vi "MotorControlMina4 with Joystick control.vi"() -> ()   [LabVIEW 2014]
uses:
  <vilib>/Utility/inputDevices.llb/joystickAcquire.vi
  <vilib>/Utility/inputDevices.llb/closeJoystick.vi
  <vilib>/DAQmx/create/channels.llb/DAQmx Create Channel (DO-Digital Output).vi
  <vilib>/DAQmx/write.llb/DAQmx Write (Digital Bool 1Line 1Point).vi
panel:
  in  "Offset (V)":dbl=5.0
  out "Oscillate Mirror? 2":bool
  out "Mirror Voltage":dbl
  in  "Oscillate Mirror?":bool
  in  "Period (s)":i32=1
  in  "Amplitude (V)":dbl=4.0
  in  "Stop":bool
  out "InstrumentMode":T1(ring)=enum."Shutdown"
  in  "XMotorRef":refnum<k7>(container)
  in  "YMotorRef":refnum<k7>(container)
  in  "ZMotorRef":refnum<k7>(container)
  out "JoystOffset":T2={"XOffset"=-99999, "YOffset"=-99999, "ZOffset"=-99999}
  out "RelJoyPos":T3
  in  "InterfaceSelector":T4(tab)
  in  "GoToTopDisp":bool
  in  "GoToBottDisp":bool
  in  "GoToExpLoc":bool
  in  "SaveTopDisp":bool
  in  "SaveBottDisp":bool
  in  "SaveExpLoc":bool
  out "Top Dispenser":T5={"X Pos (mm)"=0.5532008, "Y Pos (mm)"=0.030929338, "Z Pos (mm)"=0.77973413} {"Y Pos (mm)" format="%.3f"; "Z Pos (mm)" format="%.3f"; "X Pos (mm)" format="%.3f"}
  out "Bottom Dispenser":T5={"X Pos (mm)"=0.600309, "Y Pos (mm)"=-1.1540928, "Z Pos (mm)"=0.7938141} {"Y Pos (mm)" format="%.3f"; "Z Pos (mm)" format="%.3f"; "X Pos (mm)" format="%.3f"}
  out "Experiment Region":T5={"X Pos (mm)"=1.4278219, "Y Pos (mm)"=-0.74810517, "Z Pos (mm)"=0.7938141} {"Y Pos (mm)" format="%.3f"; "Z Pos (mm)" format="%.3f"; "X Pos (mm)" format="%.3f"}
  in  "PreviewPanel":T6(tab)
  in  "Z Motor Settings":T7={"Joyst Min Signal"=10.0, "Joyst Max Signal"=30000.0, "Vmax (mm/s)"=0.005, "Acc (mm/s/s)"=0.2, "+ JoystDirection"=2, "- JoystDirection"=1} {"Acc (mm/s/s)" format="%#.3f"; "Vmax (mm/s)" format="%#.3f"}
  in  "Y Motor Settings":T7={"Joyst Min Signal"=10.0, "Joyst Max Signal"=20000.0, "Vmax (mm/s)"=0.03, "Acc (mm/s/s)"=0.5, "+ JoystDirection"=1, "- JoystDirection"=2} {"Acc (mm/s/s)" format="%#.3f"; "Vmax (mm/s)" format="%#.3f"}
  in  "X Motor Settings":T7={"Joyst Min Signal"=10.0, "Joyst Max Signal"=20000.0, "Vmax (mm/s)"=0.03, "Acc (mm/s/s)"=0.5, "+ JoystDirection"=2, "- JoystDirection"=1} {"Acc (mm/s/s)" format="%#.3f"; "Vmax (mm/s)" format="%#.3f"}
  in  "Motor Cruise Param":T8={"X Acc (mm/s^2)"=0.3, "X Vmax (mm/s)"=0.3, "Y Acc (mm/s^2)"=0.3, "Y Vmax (mm/s)"=0.3, "Z Acc (mm/s^2)"=0.1, "Z Vmax (mm/s)"=0.1}
  in  "Motor Limits":T9={"XMin"=-0.8, "XMax"=3.0, "YMin"=-2.0, "YMax"=2.0, "ZMin"=0.0, "ZMax"=2.0}
  in  "Steerable Mirror Calibration":T10={"Hor. Scaling (nm/V)"=760.0, "Vert. Scaling (nm/V)"=760.0, "Hor. Mirr. Offset (V)"=0.0, "Vert. Mirr. Offset (V)"=0.0}
  in  "Steerable \nTrap\n(F12)":bool
  in  "Fixed\nTrap\n(F11)":bool
  in  "Align Traps Vertically":bool
  in  "MaxHorizontalTrapSeparation":bool
  out "X Motor State":T11={"Direction"=0, "Vel (mm/s)"=0.0, "IsActive?"=FALSE, "Pos (mm)"=-0.2957381} {"Pos (mm)" format="%#.3f"; "Vel (mm/s)" format="%#.4f"}
  out "Y Motor State":T11={"Direction"=0, "Vel (mm/s)"=0.0, "IsActive?"=FALSE, "Pos (mm)"=0.016441232} {"Pos (mm)" format="%#.3f"; "Vel (mm/s)" format="%#.4f"}
  out "Z Motor State":T11={"Direction"=0, "Vel (mm/s)"=0.0, "IsActive?"=FALSE, "Pos (mm)"=-0.26253498} {"Pos (mm)" format="%#.3f"; "Vel (mm/s)" format="%#.4f"}
  out "Move Z":bool
  out "Move XY":bool
  in  "MotorLoopDelay":u32=100
  in  "StopPassiveMode":bool caption="stop"
  in  "PMVertSlider(V)":dbl(slide)=0.005145263671875 scale=0.0..10.0 scale format="%#_3f"
  in  "PMHorizSlider(V)":dbl(slide)=0.0045623779296875 scale=2.0..10.0
  out "IsPassiveModeActive?":bool caption="stop"
  out "Force TrapA":cluster{"x":dbl[], "y":dbl[]}[](graph)
  out "Noise-Ext":cluster{"x":dbl[], "y":dbl[]}[](graph)
  out "Force TrapB":cluster{"x":dbl[], "y":dbl[]}[](graph)
  out "IsOffsetModeActive?":bool caption="stop"
  in  "StopOffset":bool caption="stop"
  out "IsForceExtActive?":bool=TRUE
  in  "StopForceExtension":bool caption="stop"
  # "ClpXP Optical Tweezers"
  # "Chamber Locations"
  # "Need a Button Here that would read the \nNormalized Offset and save it"
  # "Off"
  # "On"
  # "Off"
  # "On"
  # "Thorlabs Motor Status"
  # "Passive Mode"
  # "when I switch tabs from the passive mode to basic mode, the recording doesn't stop"
  # "The sliders don't do anything in passive mode, fix it"
  # "Whenever I click on Ackquire Offset, it goes back to the basic operation, then I have to ckick again"
  # "Trap Motion Control"
  # "Steerable Mirror Info"
  # "Zero-Force Offset Mode"
  # "High Frequency Data Acquisition"
  # "Adjust the length of acquisition time"
  # "Force-Extension Mode"
  # "Y"
  # "+"
  # "X"
  # "-"
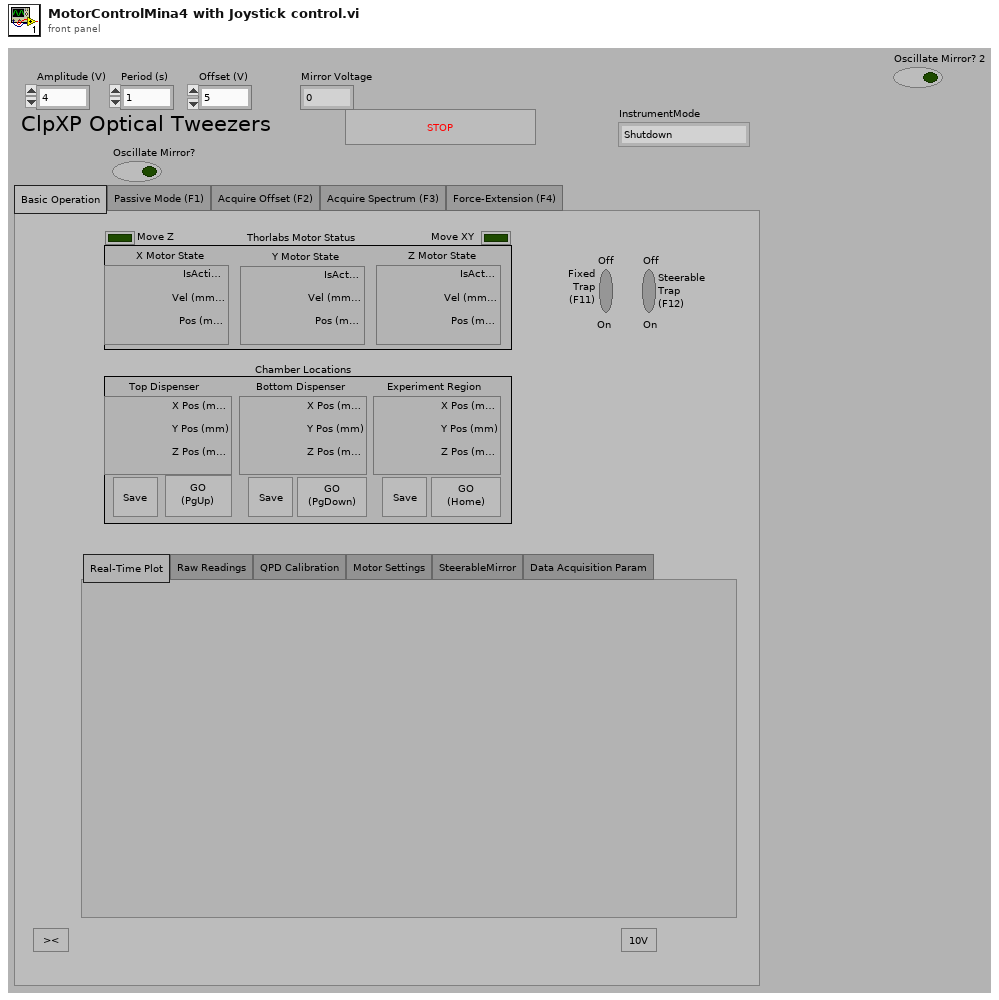
[diagram p1: front panel]
types:
  T1 = enum16{"InitializeJoystick", "InitializeMotors", "BasicMode", "PassiveMode", "AcquireOffsetMode", "AcquireSpectrumMode", "Force-ExtensionMode", "Shutdown"}
  T2 = cluster{"XOffset":i32, "YOffset":i32, "ZOffset":i32}
  T3 = cluster{"XRelPos":i32, "YRelPos":i32, "ZRelPos":i32}
  T4 = enum32{"Basic Operation", "Passive Mode (F1)", "Acquire Offset (F2)", "Acquire Spectrum (F3)", "Force-Extension (F4)"}
  T5 = cluster{"X Pos (mm)":sgl, "Y Pos (mm)":sgl, "Z Pos (mm)":sgl}
  T6 = enum32{"Real-Time Plot", "Raw Readings", "QPD Calibration", "Motor Settings", "SteerableMirror", "Data Acquisition Param"}
  T7 = cluster{"Joyst Min Signal":dbl, "Joyst Max Signal":dbl, "Vmax (mm/s)":sgl, "Acc (mm/s/s)":sgl, "+ JoystDirection":i32, "- JoystDirection":i32}
  T8 = cluster{"X Acc (mm/s^2)":sgl, "X Vmax (mm/s)":sgl, "Y Acc (mm/s^2)":sgl, "Y Vmax (mm/s)":sgl, "Z Acc (mm/s^2)":sgl, "Z Vmax (mm/s)":sgl}
  T9 = cluster{"XMin":sgl, "XMax":sgl, "YMin":sgl, "YMax":sgl, "ZMin":sgl, "ZMax":sgl}
  T10 = cluster{"Hor. Scaling (nm/V)":dbl, "Vert. Scaling (nm/V)":dbl, "Hor. Mirr. Offset (V)":dbl, "Vert. Mirr. Offset (V)":dbl}
  T11 = cluster{"Direction":i32, "Vel (mm/s)":sgl, "IsActive?":bool, "Pos (mm)":sgl}
  T12 = cluster{"XMotorRef":refnum<k7>, "YMotorRef":refnum<k7>, "ZMotorRef":refnum<k7>}
  T13 = cluster{"Motor Reference":refnum<k7>, "Motor Reference":refnum<k7>, "Motor Reference":refnum<k7>}
  T14 = cluster{"X axis":i32, "Y axis":i32, "Z axis":i32, "X axis rotation":i32, "Y axis rotation":i32, "Z axis rotation":i32, "U axis":i32, "V axis":i32}
  T15 = cluster{"button 1":bool, "button 2":bool, "button 3":bool, "button 4":bool, "button 5":bool, "button 6":bool, "button 7":bool, "button 8":bool, "button 9":bool, "button 10":bool, "button 11":bool, "button 12":bool, "button 13":bool, "button 14":bool, "button 15":bool, "button 16":bool, "button 17":bool, "button 18":bool, "button 19":bool, "button 20":bool, "button 21":bool, "button 22":bool, "button 23":bool, "button 24":bool, "button 25":bool, "button 26":bool, "button 27":bool, "button 28":bool, "button 29":bool, "button 30":bool, "button 31":bool, "button 32":bool}
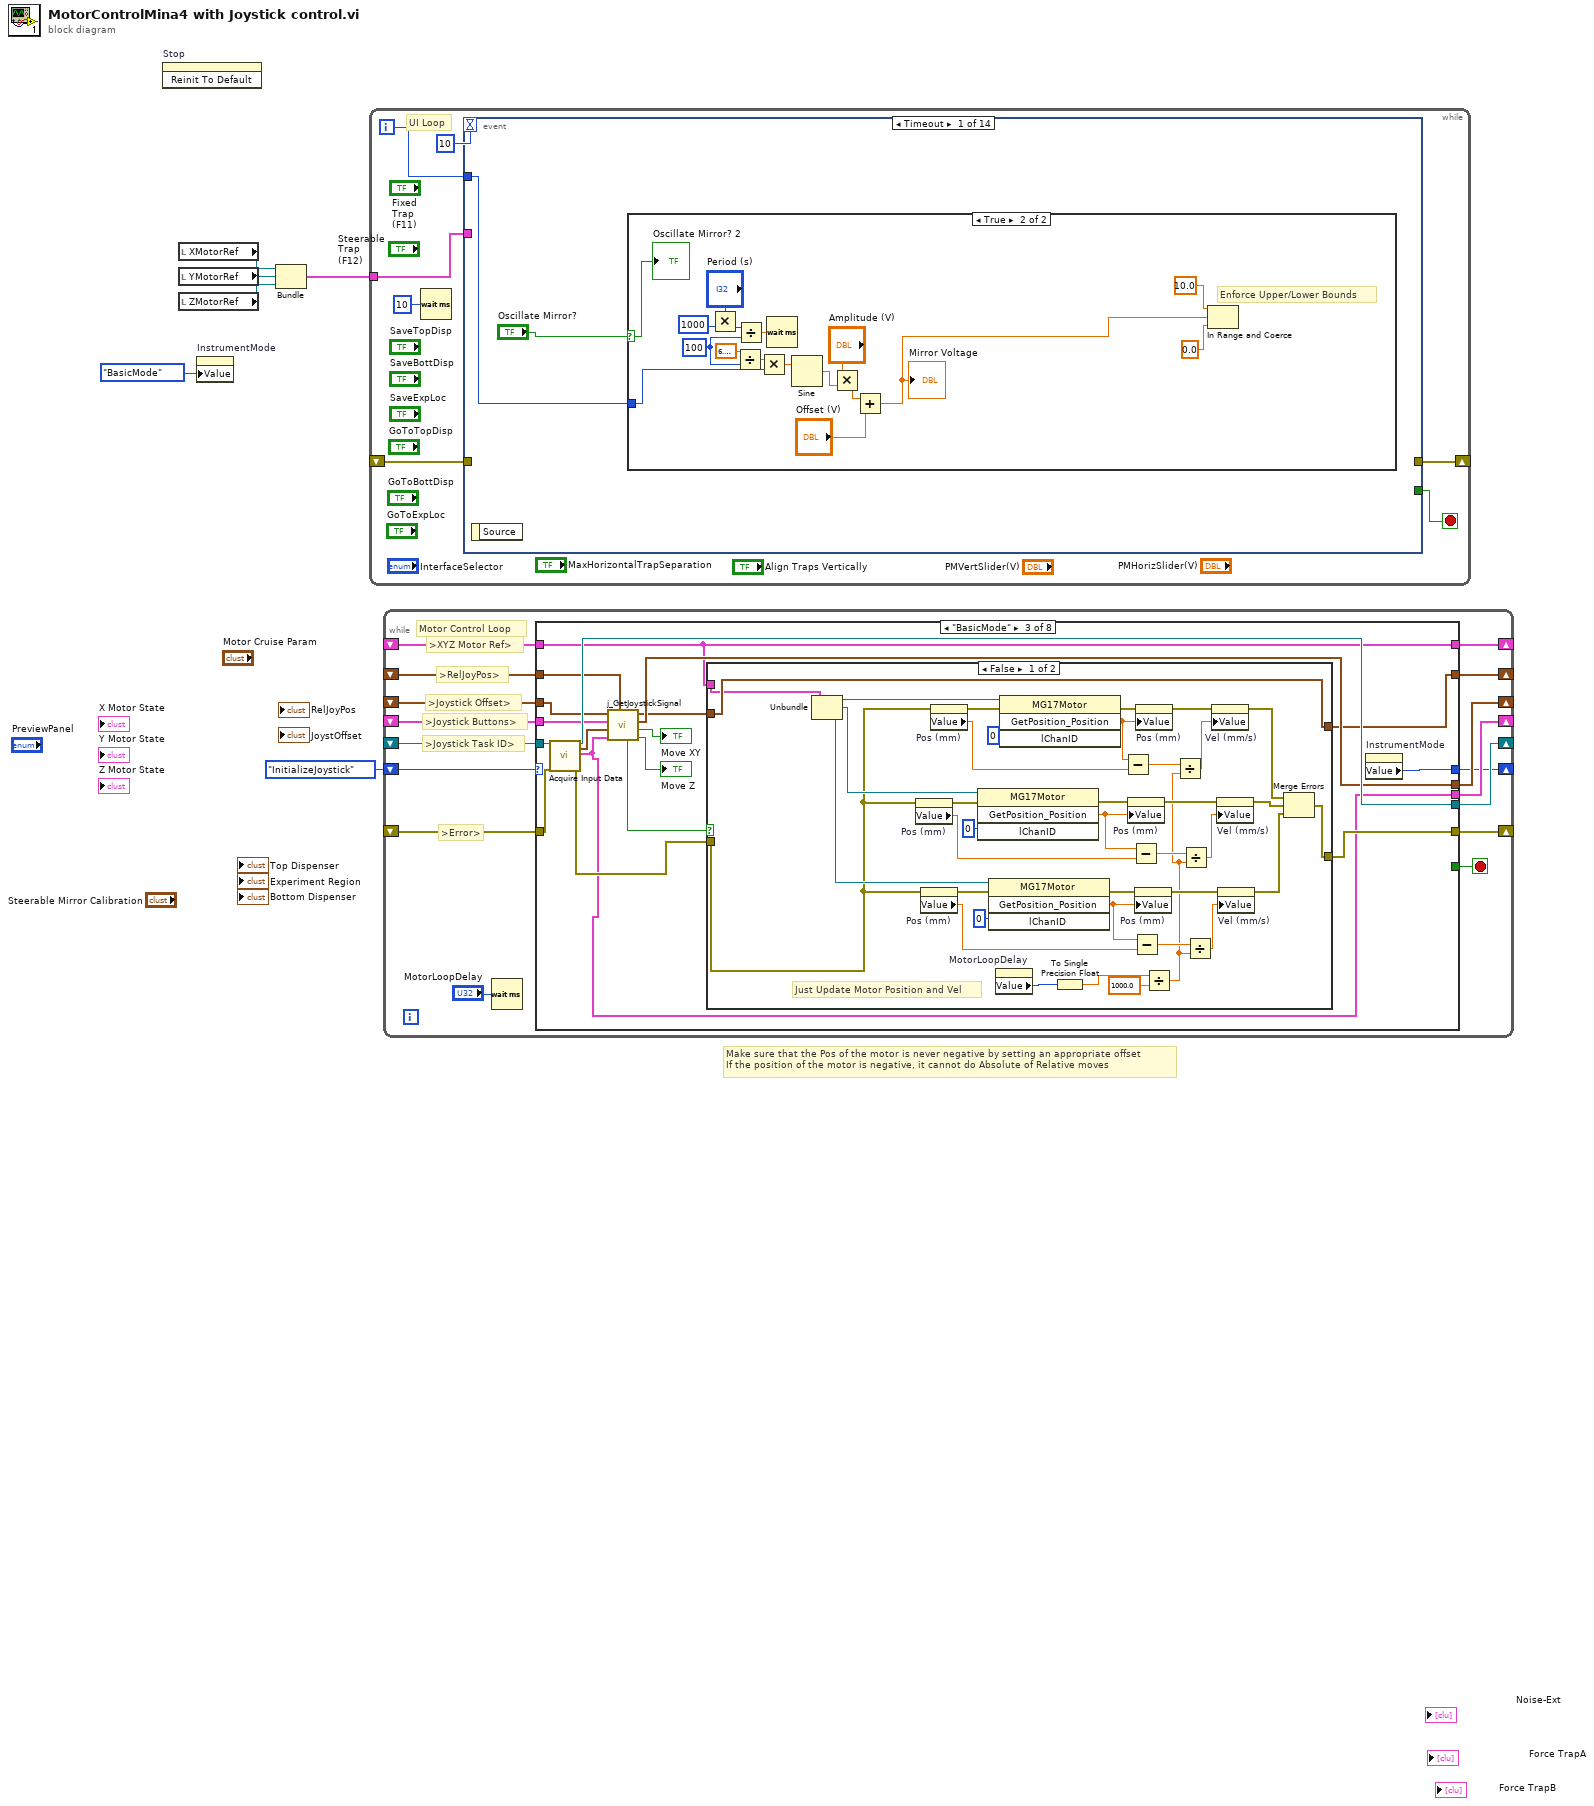
[diagram p0: block diagram]
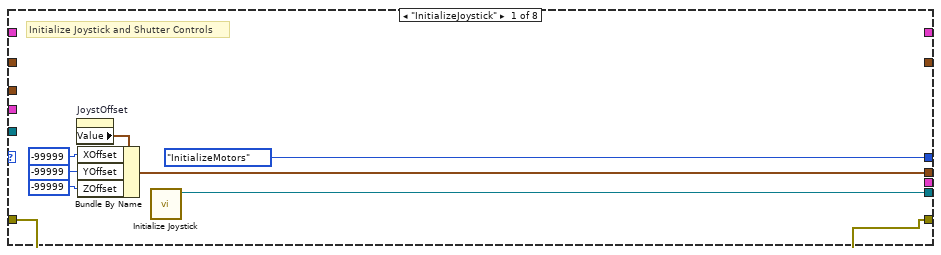
[diagram p2: hidden frame]
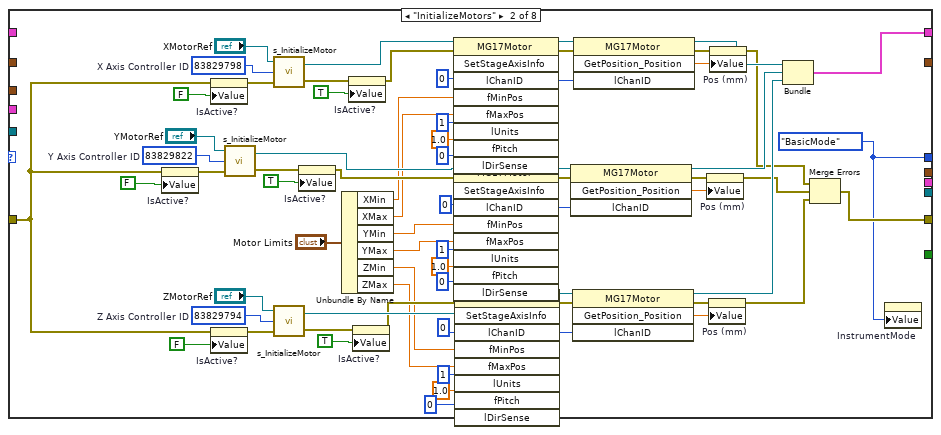
[diagram p3: hidden frame]
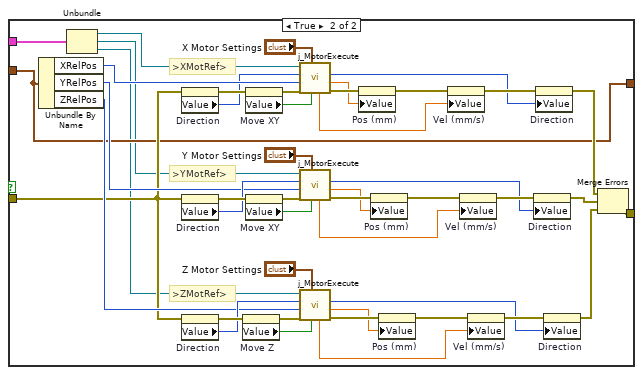
[diagram p4: hidden frame]
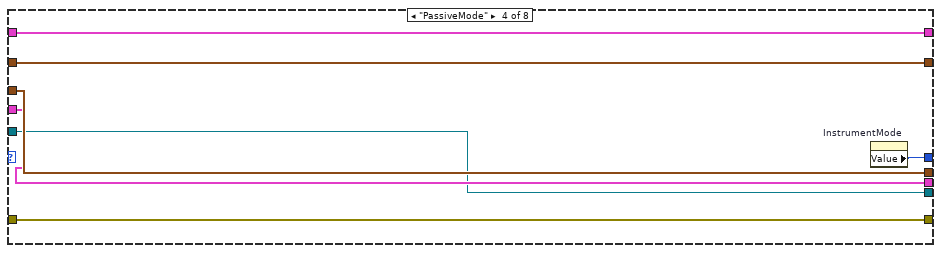
[diagram p5: hidden frame]
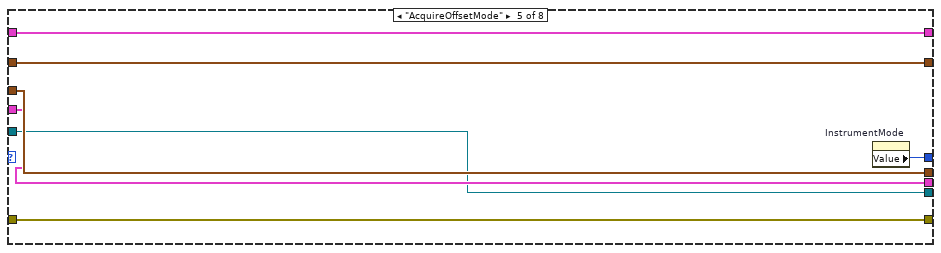
[diagram p6: hidden frame]
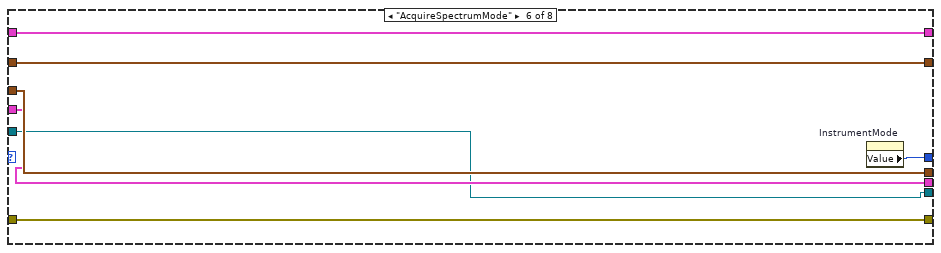
[diagram p7: hidden frame]
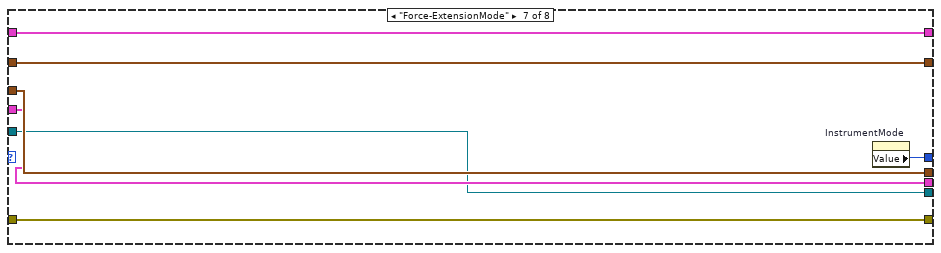
[diagram p8: hidden frame]
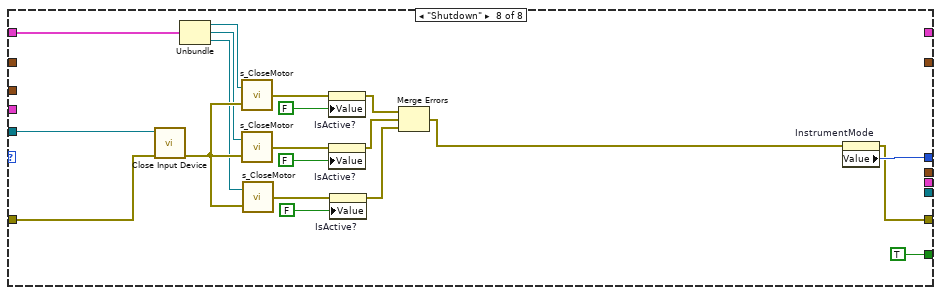
[diagram p9: hidden frame]
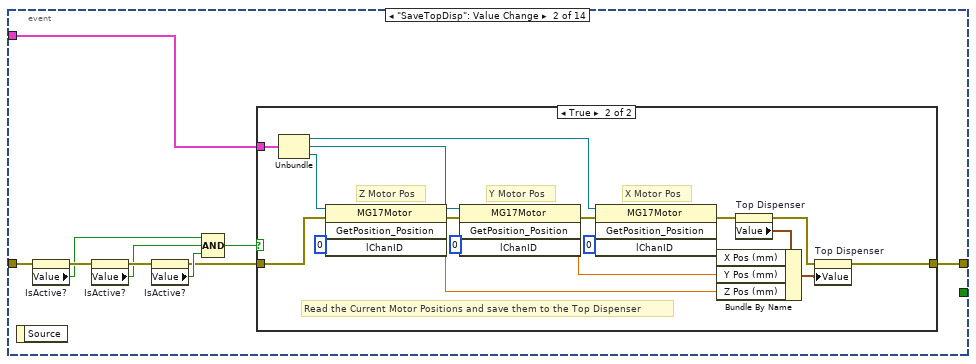
[diagram p11: hidden frame]
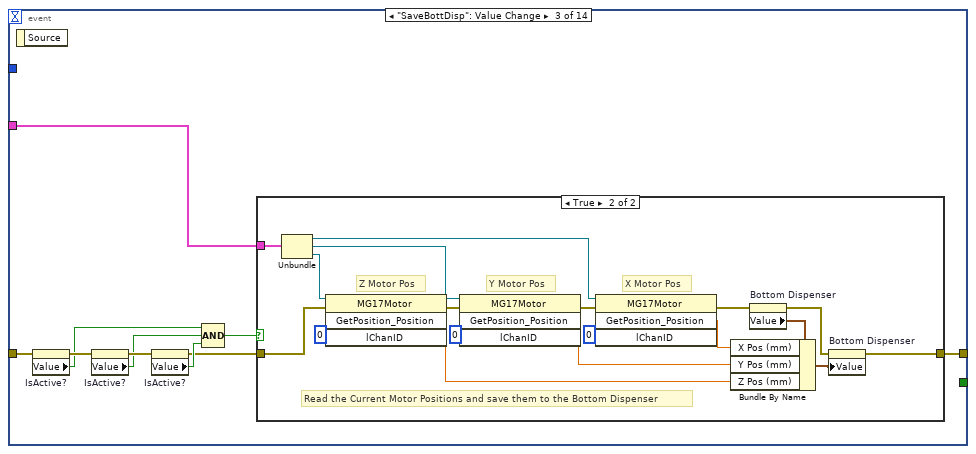
[diagram p13: hidden frame]
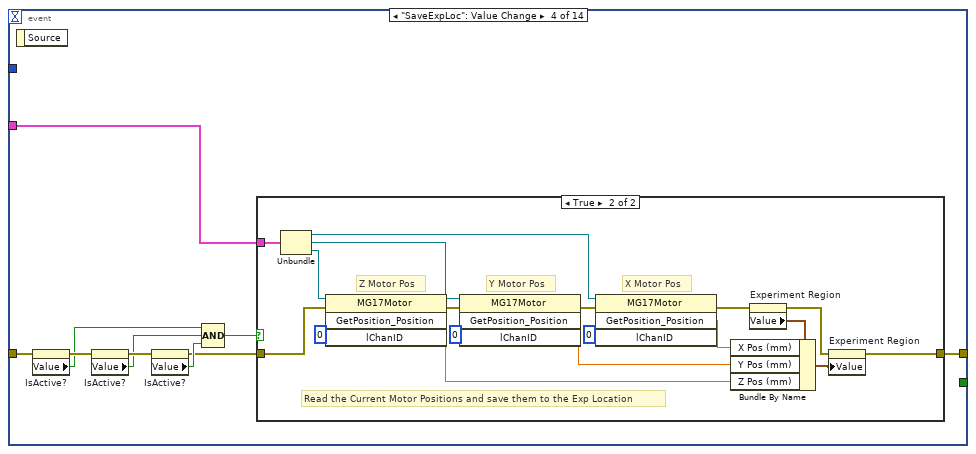
[diagram p15: hidden frame]
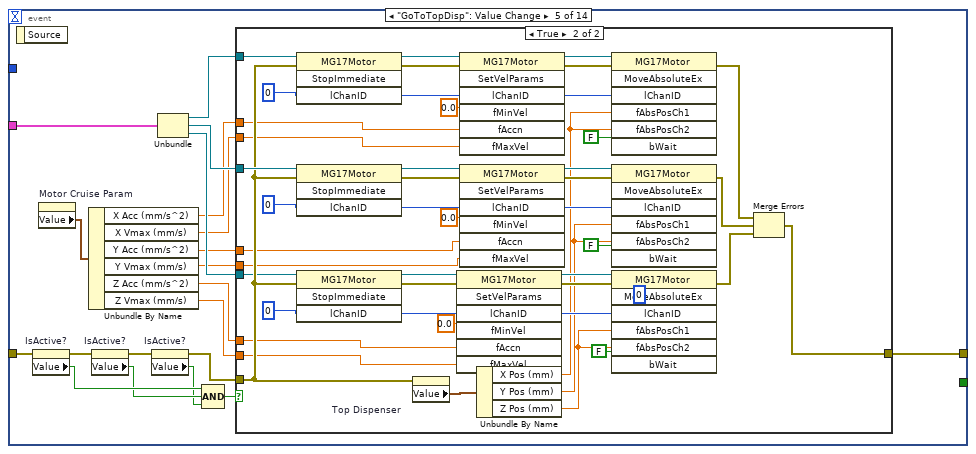
[diagram p17: hidden frame]
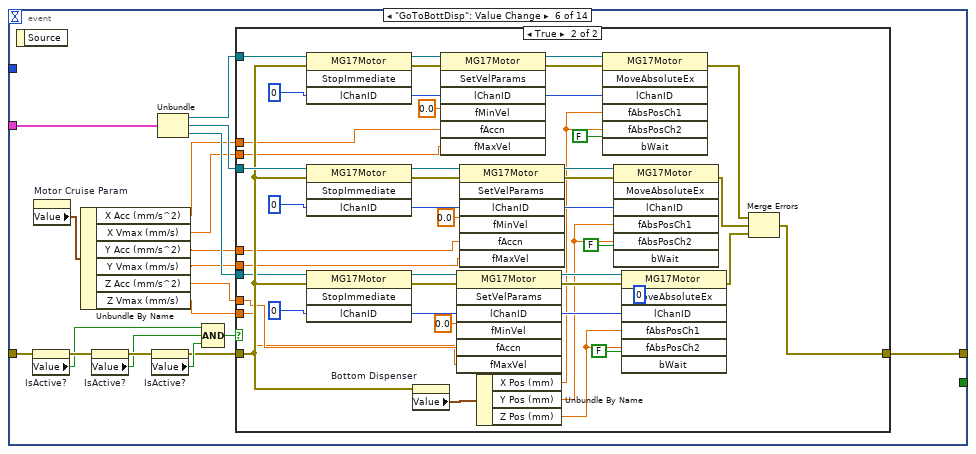
[diagram p19: hidden frame]
diagram:
  # "Make sure that the Pos of the motor is never negative by setting an appropriate offset\nIf the position of the motor is negative, it cannot do Absolute of Relative moves"
  n1 = invoke on="Stop" class="Bool" method="Reinit To Default"() -> ()  [unwired: 3 in, 3 out]
  n2 = local read "XMotorRef"() -> (w6:refnum<k7>)
  n3 = local read "YMotorRef"() -> (w5:refnum<k7>)
  n4 = local read "ZMotorRef"() -> (w4:refnum<k7>)
  n5 = property on="InstrumentMode" class="Enum (strict)"("Value"=T1."BasicMode") -> ()  [unwired: 2 in, 2 out]
  n6 = Bundle("XMotorRef"=w6, "YMotorRef"=w5, "ZMotorRef"=w4) -> (w3:T12)  [unwired: 1 in]
  n7 = while {
    shift-right: [w12] -> _
    shift-left: _ -> [w11]
    tunnel: w3 -> [w10]
    i -> [w8]
    stop <- w9 stop-if-true
    # "UI Loop"
    n8 = Wait (ms)(milliseconds to wait=u32 10) -> ()  [unwired: 1 out]
    n9 = event shown="[0] Timeout" {
      selector: _ -> [_ _ _ _ _ _ _ _ _ _ _ _ _ _]
      dyn-events: _ -> [_ _ _ _ _ _ _ _ _ _ _ _ _ _]
      timeout: 10 -> [_ _ _ _ _ _ _ _ _ _ _ _ _ _]
      tunnel: [_ w35 w64 w93 w132 w198 w264 w318 _ w329 _ _ _ w357] -> w12
      tunnel: w11 -> [_ w34 w63 w92 w131 w197 w263 w321 w328 w329 _ _ _ w357]
      tunnel: [_ _ _ _ _ _ _ _ _ _ _ _ _ "Stop"] -> w9
      tunnel: w10 -> [_ w33 w62 w91 w130 w196 w262 _ _ _ _ _ _ _]
      tunnel: w8 -> [w15 _ _ _ _ _ _ _ _ _ _ _ _ _]
      tunnel: [_ _ _ _ _ _ _ _ w328 _ _ _ _ _] -> _
      event Timeout {
        n10 = event-data() -> ()  [unwired: 1 in, 1 out]
        n11 = case shown="True" "Oscillate Mirror?" {
          selector: "Oscillate Mirror?" -> [_ w21]
          tunnel: w15 -> [_ w22]
          frame False {
          }
          frame True {
            w31 = 100
            # "Enforce Upper/Lower Bounds"
            n12 = Multiply(x="Period (s)", y=1000) -> (x*y=w29:i32)
            n13 = Divide(x=6.283185307179586, y=w31) -> (x/y=w25:dbl)
            n14 = Divide(x=w29, y=w31) -> (x/y=w30:dbl)
            n15 = Multiply(x=w25, y=w22) -> (x*y=w26:dbl)
            n16 = Wait (ms)(milliseconds to wait=w30) -> ()  [unwired: 1 out]
            n17 = Sine(x=w26) -> (sin(x)=w27:dbl)
            n18 = Multiply(x="Amplitude (V)", y=w27) -> (x*y=w19:dbl)
            n19 = Add(x=w19, y="Offset (V)") -> (x+y=w16:dbl)
            "Mirror Voltage" <- w16
            n20 = In Range and Coerce(upper limit=10.0, x=w16, lower limit=0.0 ("upper limit")) -> ()  [unwired: 2 out]
            "Oscillate Mirror? 2" <- w21
          }
        }
      }
      event "SaveTopDisp": Value Change {
        n21 = event-data() -> ()  [unwired: 1 in, 1 out]
        n22 = property on="IsActive?" class="Bool (strict)"(error in=w34) -> (error out=w42:errorcluster, "Value"=w40:bool)  [unwired: 1 in, 1 out]
        n23 = property on="IsActive?" class="Bool (strict)"(error in=w42) -> (error out=w41:errorcluster, "Value"=w39:bool)  [unwired: 1 in, 1 out]
        n24 = property on="IsActive?" class="Bool (strict)"(error in=w41) -> (error out=w36:errorcluster, "Value"=w38:bool)  [unwired: 1 in, 1 out]
        n25 = Compound Arithmetic op=AND(w40, w39, w38) -> (w37:bool)
        n26 = case shown="True" w37 {
          tunnel: w36 -> [w43 w61]
          tunnel: [w43 w48] -> w35
          tunnel: w33 -> [_ w47]
          frame False {
          }
          frame True {
            # "Read the Current Motor Positions and save them to the Top Dispenser"
            # "X Motor Pos"
            # "Y Motor Pos"
            # "Z Motor Pos"
            n27 = Unbundle(w47) -> ("XMotorRef"=w44:refnum<k7>, "YMotorRef"=w45:refnum<k7>, "ZMotorRef"=w46:refnum<k7>)
            n28 = invoke class="MG17Motor" method="GetPosition_Position"(reference=w46, error in=w61, "lChanID"=0) -> (error out=w58:errorcluster, "GetPosition_Position"=w51:sgl)  [unwired: 1 in, 2 out]
            n29 = invoke class="MG17Motor" method="GetPosition_Position"(reference=w45, error in=w58, "lChanID"=0) -> (error out=w56:errorcluster, "GetPosition_Position"=w50:sgl)  [unwired: 1 in, 2 out]
            n30 = invoke class="MG17Motor" method="GetPosition_Position"(reference=w44, error in=w56, "lChanID"=0) -> (error out=w55:errorcluster, "GetPosition_Position"=w49:sgl)  [unwired: 1 in, 2 out]
            n31 = property on="Top Dispenser" class="Clust (strict)"(error in=w55) -> (error out=w54:errorcluster, "Value"=w53:T5)  [unwired: 1 in, 1 out]
            n32 = Bundle By Name(cluster=w53, "X Pos (mm)"=w49, "Y Pos (mm)"=w50, "Z Pos (mm)"=w51) -> (w52:T5)
            n33 = property on="Top Dispenser" class="Clust (strict)"(error in=w54, "Value"=w52) -> (error out=w48:errorcluster)  [unwired: 1 in, 1 out]
          }
        }
      }
      event "SaveBottDisp": Value Change {
        n34 = event-data() -> ()  [unwired: 1 in, 1 out]
        n35 = property on="IsActive?" class="Bool (strict)"(error in=w63) -> (error out=w71:errorcluster, "Value"=w69:bool)  [unwired: 1 in, 1 out]
        n36 = property on="IsActive?" class="Bool (strict)"(error in=w71) -> (error out=w70:errorcluster, "Value"=w68:bool)  [unwired: 1 in, 1 out]
        n37 = property on="IsActive?" class="Bool (strict)"(error in=w70) -> (error out=w65:errorcluster, "Value"=w67:bool)  [unwired: 1 in, 1 out]
        n38 = Compound Arithmetic op=AND(w69, w68, w67) -> (w66:bool)
        n39 = case shown="True" w66 {
          tunnel: w65 -> [w72 w90]
          tunnel: [w72 w77] -> w64
          tunnel: w62 -> [_ w76]
          frame False {
          }
          frame True {
            # "Read the Current Motor Positions and save them to the Bottom Dispenser"
            # "X Motor Pos"
            # "Y Motor Pos"
            # "Z Motor Pos"
            n40 = Unbundle(w76) -> ("XMotorRef"=w73:refnum<k7>, "YMotorRef"=w74:refnum<k7>, "ZMotorRef"=w75:refnum<k7>)
            n41 = invoke class="MG17Motor" method="GetPosition_Position"(reference=w75, error in=w90, "lChanID"=0) -> (error out=w87:errorcluster, "GetPosition_Position"=w80:sgl)  [unwired: 1 in, 2 out]
            n42 = invoke class="MG17Motor" method="GetPosition_Position"(reference=w74, error in=w87, "lChanID"=0) -> (error out=w85:errorcluster, "GetPosition_Position"=w79:sgl)  [unwired: 1 in, 2 out]
            n43 = invoke class="MG17Motor" method="GetPosition_Position"(reference=w73, error in=w85, "lChanID"=0) -> (error out=w84:errorcluster, "GetPosition_Position"=w78:sgl)  [unwired: 1 in, 2 out]
            n44 = property on="Bottom Dispenser" class="Clust (strict)"(error in=w84) -> (error out=w83:errorcluster, "Value"=w82:T5)  [unwired: 1 in, 1 out]
            n45 = Bundle By Name(cluster=w82, "X Pos (mm)"=w78, "Y Pos (mm)"=w79, "Z Pos (mm)"=w80) -> (w81:T5)
            n46 = property on="Bottom Dispenser" class="Clust (strict)"(error in=w83, "Value"=w81) -> (error out=w77:errorcluster)  [unwired: 1 in, 1 out]
          }
        }
      }
      event "SaveExpLoc": Value Change {
        n47 = event-data() -> ()  [unwired: 1 in, 1 out]
        n48 = property on="IsActive?" class="Bool (strict)"(error in=w92) -> (error out=w100:errorcluster, "Value"=w98:bool)  [unwired: 1 in, 1 out]
        n49 = property on="IsActive?" class="Bool (strict)"(error in=w100) -> (error out=w99:errorcluster, "Value"=w97:bool)  [unwired: 1 in, 1 out]
        n50 = property on="IsActive?" class="Bool (strict)"(error in=w99) -> (error out=w94:errorcluster, "Value"=w96:bool)  [unwired: 1 in, 1 out]
        n51 = Compound Arithmetic op=AND(w98, w97, w96) -> (w95:bool)
        n52 = case shown="True" w95 {
          tunnel: w94 -> [w101 w119]
          tunnel: [w101 w106] -> w93
          tunnel: w91 -> [_ w105]
          frame False {
          }
          frame True {
            # "Read the Current Motor Positions and save them to the Exp Location"
            # "X Motor Pos"
            # "Y Motor Pos"
            # "Z Motor Pos"
            n53 = Unbundle(w105) -> ("XMotorRef"=w102:refnum<k7>, "YMotorRef"=w103:refnum<k7>, "ZMotorRef"=w104:refnum<k7>)
            n54 = invoke class="MG17Motor" method="GetPosition_Position"(reference=w104, error in=w119, "lChanID"=0) -> (error out=w116:errorcluster, "GetPosition_Position"=w109:sgl)  [unwired: 1 in, 2 out]
            n55 = invoke class="MG17Motor" method="GetPosition_Position"(reference=w103, error in=w116, "lChanID"=0) -> (error out=w114:errorcluster, "GetPosition_Position"=w108:sgl)  [unwired: 1 in, 2 out]
            n56 = invoke class="MG17Motor" method="GetPosition_Position"(reference=w102, error in=w114, "lChanID"=0) -> (error out=w113:errorcluster, "GetPosition_Position"=w107:sgl)  [unwired: 1 in, 2 out]
            n57 = property on="Experiment Region" class="Clust (strict)"(error in=w113) -> (error out=w112:errorcluster, "Value"=w111:T5)  [unwired: 1 in, 1 out]
            n58 = Bundle By Name(cluster=w111, "X Pos (mm)"=w107, "Y Pos (mm)"=w108, "Z Pos (mm)"=w109) -> (w110:T5)
            n59 = property on="Experiment Region" class="Clust (strict)"(error in=w112, "Value"=w110) -> (error out=w106:errorcluster)  [unwired: 1 in, 1 out]
          }
        }
      }
      event "GoToTopDisp": Value Change {
        n60 = event-data() -> ()  [unwired: 1 in, 1 out]
        n61 = property on="IsActive?" class="Bool (strict)"(error in=w131) -> (error out=w139:errorcluster, "Value"=w137:bool)  [unwired: 1 in, 1 out]
        n62 = property on="Motor Cruise Param" class="Clust (strict)"() -> ("Value"=w120:T8)  [unwired: 2 in, 2 out]
        n63 = Unbundle By Name(w120) -> ("X Acc (mm/s^2)"=w124:sgl, "X Vmax (mm/s)"=w123:sgl, "Y Acc (mm/s^2)"=w122:sgl, "Y Vmax (mm/s)"=w121:sgl, "Z Acc (mm/s^2)"=w126:sgl, "Z Vmax (mm/s)"=w125:sgl)
        n64 = property on="IsActive?" class="Bool (strict)"(error in=w139) -> (error out=w138:errorcluster, "Value"=w136:bool)  [unwired: 1 in, 1 out]
        n65 = property on="IsActive?" class="Bool (strict)"(error in=w138) -> (error out=w133:errorcluster, "Value"=w135:bool)  [unwired: 1 in, 1 out]
        n66 = Unbundle(w130) -> ("XMotorRef"=w129:refnum<k7>, "YMotorRef"=w128:refnum<k7>, "ZMotorRef"=w127:refnum<k7>)
        n67 = Compound Arithmetic op=AND(w137, w136, w135) -> (w134:bool)
        n68 = case shown="True" w134 {
          tunnel: w133 -> [w140 w160]
          tunnel: [w140 w156] -> w132
          tunnel: w129 -> [_ w183]
          tunnel: w128 -> [_ w168]
          tunnel: w127 -> [_ w155]
          tunnel: w126 -> [_ w146]
          tunnel: w125 -> [_ w145]
          tunnel: w124 -> [_ w144]
          tunnel: w123 -> [_ w143]
          tunnel: w122 -> [_ w142]
          tunnel: w121 -> [_ w141]
          frame False {
          }
          frame True {
            (unwired) 0 ("lChanID")
            n69 = invoke class="MG17Motor" method="StopImmediate"(reference=w183, error in=w160, "lChanID"=0) -> (reference out=w181:refnum<k7>, error out=w182:errorcluster, "lChanID"=w151:i32)  [unwired: 1 in, 1 out]
            n70 = invoke class="MG17Motor" method="StopImmediate"(reference=w168, error in=w160, "lChanID"=0) -> (reference out=w175:refnum<k7>, error out=w176:errorcluster, "lChanID"=w152:i32)  [unwired: 1 in, 1 out]
            n71 = invoke class="MG17Motor" method="StopImmediate"(reference=w155, error in=w160, "lChanID"=0) -> (reference out=w165:refnum<k7>, error out=w166:errorcluster, "lChanID"=w153:i32)  [unwired: 1 in, 1 out]
            n72 = property on="Top Dispenser" class="Clust (strict)"(error in=w160) -> ("Value"=w185:T5)  [unwired: 1 in, 2 out]
            n73 = invoke class="MG17Motor" method="SetVelParams"(reference=w165, error in=w166, "lChanID"=w153, "fMinVel"=sgl 0.0, "fAccn"=w146, "fMaxVel"=w145) -> (reference out=w164:refnum<k7>, error out=w163:errorcluster, "lChanID"=w162:i32)  [unwired: 1 in, 4 out]
            n74 = invoke class="MG17Motor" method="SetVelParams"(reference=w181, error in=w182, "lChanID"=w151, "fMinVel"=sgl 0.0, "fAccn"=w144, "fMaxVel"=w143) -> (reference out=w180:refnum<k7>, error out=w179:errorcluster, "lChanID"=w178:i32)  [unwired: 1 in, 4 out]
            n75 = invoke class="MG17Motor" method="SetVelParams"(reference=w175, error in=w176, "lChanID"=w152, "fMinVel"=sgl 0.0, "fAccn"=w142, "fMaxVel"=w141) -> (reference out=w173:refnum<k7>, error out=w172:errorcluster, "lChanID"=w171:i32)  [unwired: 1 in, 4 out]
            n76 = Unbundle By Name(w185) -> ("X Pos (mm)"=w149:sgl, "Y Pos (mm)"=w148:sgl, "Z Pos (mm)"=w147:sgl)
            n77 = invoke class="MG17Motor" method="MoveAbsoluteEx"(reference=w180, error in=w179, "lChanID"=w178, "fAbsPosCh1"=w149, "fAbsPosCh2"=w149, "bWait"=FALSE) -> (error out=w159:errorcluster)  [unwired: 1 in, 6 out]
            n78 = invoke class="MG17Motor" method="MoveAbsoluteEx"(reference=w173, error in=w172, "lChanID"=w171, "fAbsPosCh1"=w148, "fAbsPosCh2"=w148, "bWait"=FALSE) -> (error out=w158:errorcluster)  [unwired: 1 in, 6 out]
            n79 = invoke class="MG17Motor" method="MoveAbsoluteEx"(reference=w164, error in=w163, "lChanID"=w162, "fAbsPosCh1"=w147, "fAbsPosCh2"=w147, "bWait"=FALSE) -> (error out=w157:errorcluster)  [unwired: 1 in, 6 out]
            n80 = Merge Errors(w159, w158, w157) -> (w156:errorcluster)
          }
        }
      }
      event "GoToBottDisp": Value Change {
        n81 = event-data() -> ()  [unwired: 1 in, 1 out]
        n82 = property on="IsActive?" class="Bool (strict)"(error in=w197) -> (error out=w205:errorcluster, "Value"=w203:bool)  [unwired: 1 in, 1 out]
        n83 = property on="Motor Cruise Param" class="Clust (strict)"() -> ("Value"=w192:T8)  [unwired: 2 in, 2 out]
        n84 = Unbundle By Name(w192) -> ("X Acc (mm/s^2)"=w191:sgl, "X Vmax (mm/s)"=w190:sgl, "Y Acc (mm/s^2)"=w189:sgl, "Y Vmax (mm/s)"=w188:sgl, "Z Acc (mm/s^2)"=w187:sgl, "Z Vmax (mm/s)"=w186:sgl)
        n85 = property on="IsActive?" class="Bool (strict)"(error in=w205) -> (error out=w204:errorcluster, "Value"=w202:bool)  [unwired: 1 in, 1 out]
        n86 = property on="IsActive?" class="Bool (strict)"(error in=w204) -> (error out=w199:errorcluster, "Value"=w201:bool)  [unwired: 1 in, 1 out]
        n87 = Unbundle(w196) -> ("XMotorRef"=w195:refnum<k7>, "YMotorRef"=w194:refnum<k7>, "ZMotorRef"=w193:refnum<k7>)
        n88 = Compound Arithmetic op=AND(w203, w202, w201) -> (w200:bool)
        n89 = case shown="True" w200 {
          tunnel: w199 -> [w206 w226]
          tunnel: [w206 w222] -> w198
          tunnel: w195 -> [_ w249]
          tunnel: w194 -> [_ w234]
          tunnel: w193 -> [_ w221]
          tunnel: w191 -> [_ w212]
          tunnel: w190 -> [_ w211]
          tunnel: w189 -> [_ w210]
          tunnel: w188 -> [_ w209]
          tunnel: w187 -> [_ w208]
          tunnel: w186 -> [_ w207]
          frame False {
          }
          frame True {
            (unwired) 0 ("lChanID")
            n90 = invoke class="MG17Motor" method="StopImmediate"(reference=w249, error in=w226, "lChanID"=0) -> (reference out=w247:refnum<k7>, error out=w248:errorcluster, "lChanID"=w217:i32)  [unwired: 1 in, 1 out]
            n91 = invoke class="MG17Motor" method="StopImmediate"(reference=w234, error in=w226, "lChanID"=0) -> (reference out=w241:refnum<k7>, error out=w242:errorcluster, "lChanID"=w218:i32)  [unwired: 1 in, 1 out]
            n92 = invoke class="MG17Motor" method="StopImmediate"(reference=w221, error in=w226, "lChanID"=0) -> (reference out=w231:refnum<k7>, error out=w232:errorcluster, "lChanID"=w219:i32)  [unwired: 1 in, 1 out]
            n93 = property on="Bottom Dispenser" class="Clust (strict)"(error in=w226) -> ("Value"=w251:T5)  [unwired: 1 in, 2 out]
            n94 = invoke class="MG17Motor" method="SetVelParams"(reference=w247, error in=w248, "lChanID"=w217, "fMinVel"=sgl 0.0, "fAccn"=w212, "fMaxVel"=w211) -> (reference out=w246:refnum<k7>, error out=w245:errorcluster, "lChanID"=w244:i32)  [unwired: 1 in, 4 out]
            n95 = invoke class="MG17Motor" method="SetVelParams"(reference=w231, error in=w232, "lChanID"=w219, "fMinVel"=sgl 0.0, "fAccn"=w208, "fMaxVel"=w207) -> (reference out=w230:refnum<k7>, error out=w229:errorcluster, "lChanID"=w228:i32)  [unwired: 1 in, 4 out]
            n96 = invoke class="MG17Motor" method="SetVelParams"(reference=w241, error in=w242, "lChanID"=w218, "fMinVel"=sgl 0.0, "fAccn"=w210, "fMaxVel"=w209) -> (reference out=w239:refnum<k7>, error out=w238:errorcluster, "lChanID"=w237:i32)  [unwired: 1 in, 4 out]
            n97 = Unbundle By Name(w251) -> ("X Pos (mm)"=w215:sgl, "Y Pos (mm)"=w214:sgl, "Z Pos (mm)"=w213:sgl)
            n98 = invoke class="MG17Motor" method="MoveAbsoluteEx"(reference=w246, error in=w245, "lChanID"=w244, "fAbsPosCh1"=w215, "fAbsPosCh2"=w215, "bWait"=FALSE) -> (error out=w225:errorcluster)  [unwired: 1 in, 6 out]
            n99 = invoke class="MG17Motor" method="MoveAbsoluteEx"(reference=w239, error in=w238, "lChanID"=w237, "fAbsPosCh1"=w214, "fAbsPosCh2"=w214, "bWait"=FALSE) -> (error out=w224:errorcluster)  [unwired: 1 in, 6 out]
            n100 = invoke class="MG17Motor" method="MoveAbsoluteEx"(reference=w230, error in=w229, "lChanID"=w228, "fAbsPosCh1"=w213, "fAbsPosCh2"=w213, "bWait"=FALSE) -> (error out=w223:errorcluster)  [unwired: 1 in, 6 out]
            n101 = Merge Errors(w225, w224, w223) -> (w222:errorcluster)
          }
        }
      }
      event "GoToExpLoc": Value Change {
        n102 = event-data() -> ()  [unwired: 1 in, 1 out]
        n103 = property on="Motor Cruise Param" class="Clust (strict)"() -> ("Value"=w258:T8)  [unwired: 2 in, 2 out]
        n104 = property on="IsActive?" class="Bool (strict)"(error in=w263) -> (error out=w271:errorcluster, "Value"=w269:bool)  [unwired: 1 in, 1 out]
        n105 = Unbundle By Name(w258) -> ("X Acc (mm/s^2)"=w257:sgl, "X Vmax (mm/s)"=w256:sgl, "Y Acc (mm/s^2)"=w255:sgl, "Y Vmax (mm/s)"=w254:sgl, "Z Acc (mm/s^2)"=w253:sgl, "Z Vmax (mm/s)"=w252:sgl)
        n106 = property on="IsActive?" class="Bool (strict)"(error in=w271) -> (error out=w270:errorcluster, "Value"=w268:bool)  [unwired: 1 in, 1 out]
        n107 = property on="IsActive?" class="Bool (strict)"(error in=w270) -> (error out=w265:errorcluster, "Value"=w267:bool)  [unwired: 1 in, 1 out]
        n108 = Unbundle(w262) -> ("XMotorRef"=w261:refnum<k7>, "YMotorRef"=w260:refnum<k7>, "ZMotorRef"=w259:refnum<k7>)
        n109 = Compound Arithmetic op=AND(w269, w268, w267) -> (w266:bool)
        n110 = case shown="True" w266 {
          tunnel: w265 -> [w272 w292]
          tunnel: [w272 w288] -> w264
          tunnel: w261 -> [_ w315]
          tunnel: w260 -> [_ w300]
          tunnel: w259 -> [_ w287]
          tunnel: w257 -> [_ w278]
          tunnel: w256 -> [_ w277]
          tunnel: w255 -> [_ w276]
          tunnel: w254 -> [_ w275]
          tunnel: w253 -> [_ w274]
          tunnel: w252 -> [_ w273]
          frame False {
          }
          frame True {
            (unwired) 0 ("lChanID")
            n111 = invoke class="MG17Motor" method="StopImmediate"(reference=w315, error in=w292, "lChanID"=0) -> (reference out=w313:refnum<k7>, error out=w314:errorcluster, "lChanID"=w283:i32)  [unwired: 1 in, 1 out]
            n112 = invoke class="MG17Motor" method="StopImmediate"(reference=w300, error in=w292, "lChanID"=0) -> (reference out=w307:refnum<k7>, error out=w308:errorcluster, "lChanID"=w284:i32)  [unwired: 1 in, 1 out]
            n113 = invoke class="MG17Motor" method="StopImmediate"(reference=w287, error in=w292, "lChanID"=0) -> (reference out=w297:refnum<k7>, error out=w298:errorcluster, "lChanID"=w285:i32)  [unwired: 1 in, 1 out]
            n114 = property on="Experiment Region" class="Clust (strict)"(error in=w292) -> ("Value"=w317:T5)  [unwired: 1 in, 2 out]
            n115 = invoke class="MG17Motor" method="SetVelParams"(reference=w313, error in=w314, "lChanID"=w283, "fMinVel"=sgl 0.0, "fAccn"=w278, "fMaxVel"=w277) -> (reference out=w312:refnum<k7>, error out=w311:errorcluster, "lChanID"=w310:i32)  [unwired: 1 in, 4 out]
            n116 = invoke class="MG17Motor" method="SetVelParams"(reference=w297, error in=w298, "lChanID"=w285, "fMinVel"=sgl 0.0, "fAccn"=w274, "fMaxVel"=w273) -> (reference out=w296:refnum<k7>, error out=w295:errorcluster, "lChanID"=w294:i32)  [unwired: 1 in, 4 out]
            n117 = invoke class="MG17Motor" method="SetVelParams"(reference=w307, error in=w308, "lChanID"=w284, "fMinVel"=sgl 0.0, "fAccn"=w276, "fMaxVel"=w275) -> (reference out=w305:refnum<k7>, error out=w304:errorcluster, "lChanID"=w303:i32)  [unwired: 1 in, 4 out]
            n118 = Unbundle By Name(w317) -> ("X Pos (mm)"=w281:sgl, "Y Pos (mm)"=w280:sgl, "Z Pos (mm)"=w279:sgl)
            n119 = invoke class="MG17Motor" method="MoveAbsoluteEx"(reference=w312, error in=w311, "lChanID"=w310, "fAbsPosCh1"=w281, "fAbsPosCh2"=w281, "bWait"=FALSE) -> (error out=w291:errorcluster)  [unwired: 1 in, 6 out]
            n120 = invoke class="MG17Motor" method="MoveAbsoluteEx"(reference=w305, error in=w304, "lChanID"=w303, "fAbsPosCh1"=w280, "fAbsPosCh2"=w280, "bWait"=FALSE) -> (error out=w290:errorcluster)  [unwired: 1 in, 6 out]
            n121 = invoke class="MG17Motor" method="MoveAbsoluteEx"(reference=w296, error in=w295, "lChanID"=w294, "fAbsPosCh1"=w279, "fAbsPosCh2"=w279, "bWait"=FALSE) -> (error out=w289:errorcluster)  [unwired: 1 in, 6 out]
            n122 = Merge Errors(w291, w290, w289) -> (w288:errorcluster)
          }
        }
      }
      event "Steerable \nTrap\n(F12)": Value Change {
        # "Update the TTL signal to the shutter"
        n123 = event-data() -> ("NewVal"=w323:bool)  [unwired: 1 in]
        n124 = call-poly <vilib>:"DAQmx Create Virtual Channel.vi"("lines"=tag "PCI-6036E/port0/line0", "name to assign"="TrapA_TTL_Signal", "error in"=w321) -> ("task out"=w325:refnum<k21>, "error out"=w322:errorcluster)  [unwired: 11 in]
        n125 = call-poly <vilib>:"DAQmx Write.vi"("task/channels in"=w325, "data"=w323, "timeout"=10.0, "error in"=w322) -> ("task out"=w320:refnum<k21>, "error out"=w319:errorcluster)  [unwired: 9 in, 1 out]
        n126 = call <vilib>:"DAQmx Clear Task.vi"("task in"=w320, "error in"=w319) -> ("error out"=w318:errorcluster)  [unwired: 13 in]
      }
      event "Fixed\nTrap\n(F11)": Value Change {
        n127 = event-data() -> ()  [unwired: 1 in, 1 out]
      }
      event "InterfaceSelector": Value Change {
        n128 = event-data() -> ("NewVal"=w331:T4)  [unwired: 1 in]
        n129 = case shown="\"Force-Extension (F4)\"" w331 {
          tunnel: [T1."BasicMode" T1."PassiveMode" T1."AcquireOffsetMode" T1."AcquireSpectrumMode" T1."Force-ExtensionMode"] -> w330
          frame "Basic Operation" {
          }
          frame "Passive Mode (F1)" {
            n130 = property on="IsPassiveModeActive?" class="Bool (strict)"("Value"=TRUE ("StopOffset")) -> ()  [unwired: 2 in, 2 out]
          }
          frame "Acquire Offset (F2)" {
            n131 = property on="IsOffsetModeActive?" class="Bool (strict)"("Value"=TRUE ("StopOffset")) -> ()  [unwired: 2 in, 2 out]
          }
          frame "Acquire Spectrum (F3)" {
          }
          frame "Force-Extension (F4)" {
            n132 = property on="IsForceExtActive?" class="Bool (strict)"("Value"=TRUE ("StopOffset")) -> ()  [unwired: 2 in, 2 out]
          }
        }
        "InstrumentMode" <- w330
      }
      event "StopOffset": Value Change {
        n133 = event-data() -> ("NewVal"=w340:bool)  [unwired: 1 in, 5 out]
        n134 = case shown="True" w340 {
          frame False {
          }
          frame True {
            n135 = flat-sequence {
              frame #0 {
                n136 = Not(x="StopOffset") -> (.not. x?=→"IsOffsetModeActive?":bool)
              }
              frame #1 {
                n137 = property on="InterfaceSelector" class="TabCtl (strict)"("Value"=T4."Basic Operation" ("InterfaceSelector")) -> ()  [unwired: 2 in, 2 out]
                n138 = property on="InstrumentMode" class="Enum (strict)"("Value"=T1."BasicMode" ("InstrumentMode")) -> ()  [unwired: 2 in, 2 out]
              }
            }
          }
        }
      }
      event "StopPassiveMode": Value Change {
        n139 = event-data() -> ("NewVal"=w345:bool)  [unwired: 1 in, 5 out]
        n140 = case shown="True" w345 {
          frame False {
          }
          frame True {
            n141 = flat-sequence {
              frame #0 {
                n142 = Not(x="StopPassiveMode") -> (.not. x?=→"IsPassiveModeActive?":bool)
              }
              frame #1 {
                n143 = property on="InterfaceSelector" class="TabCtl (strict)"("Value"=T4."Basic Operation" ("InterfaceSelector")) -> ()  [unwired: 2 in, 2 out]
                n144 = property on="InstrumentMode" class="Enum (strict)"("Value"=T1."BasicMode" ("InstrumentMode")) -> ()  [unwired: 2 in, 2 out]
              }
            }
          }
        }
      }
      event "StopForceExtension": Value Change {
        n145 = event-data() -> ("NewVal"=w350:bool)  [unwired: 1 in, 5 out]
        n146 = case shown="True" w350 {
          frame False {
          }
          frame True {
            n147 = flat-sequence {
              frame #0 {
                n148 = Not(x="StopForceExtension") -> (.not. x?=→"IsForceExtActive?":bool)
              }
              frame #1 {
                n149 = property on="InterfaceSelector" class="TabCtl (strict)"("Value"=T4."Basic Operation" ("InterfaceSelector")) -> ()  [unwired: 2 in, 2 out]
                n150 = property on="InstrumentMode" class="Enum (strict)"("Value"=T1."BasicMode" ("InstrumentMode")) -> ()  [unwired: 2 in, 2 out]
              }
            }
          }
        }
      }
      event "Stop": Value Change {
        n151 = event-data() -> ()  [unwired: 1 in, 1 out]
        n152 = property on="InstrumentMode" class="Enum (strict)"("Value"=T1."Shutdown") -> ()  [unwired: 2 in, 2 out]
      }
    }
  }
  n153 = while {
    shift-right: [w359] -> _
    shift-left: T1."InitializeJoystick" -> [w358]
    shift-right: [w373] -> _
    shift-left: _ -> [w366]
    shift-right: [w370] -> _
    shift-left: _ -> [w372]
    shift-right: [w371] -> _
    shift-left: _ -> [w369]
    shift-right: [w368] -> _
    shift-left: _ -> [w367]
    shift-right: [w365] -> _
    shift-left: _ -> [w362]
    shift-right: [w363] -> _
    shift-left: _ -> [w364]
    stop <- w360 stop-if-true
    # "Motor Control Loop"
    # ">Joystick Offset>"
    # ">RelJoyPos>"
    # ">XYZ Motor Ref>"
    # ">Error>"
    # ">Joystick Task ID>"
    # ">Joystick Buttons>"
    n154 = Wait (ms)(milliseconds to wait="MotorLoopDelay") -> ()  [unwired: 1 out]
    n155 = case shown="\"BasicMode\"" w358 {
      tunnel: [w378 _ w464 w554 w561 w568 w575 _] -> w373
      tunnel: [T1."InitializeMotors" w382 w453 w558 w565 w572 w579 w598] -> w359
      tunnel: w372 -> [w374 w431 w466 w557 w564 w571 w578 w583]
      tunnel: [w377 _ w465 w552 w559 w566 w573 _] -> w371
      tunnel: [w374 w430 w457 w557 w564 w571 w578 w580] -> w370
      tunnel: w369 -> [_ _ w467 w552 w559 w566 w573 w582]
      tunnel: [_ _ w451 w553 w560 w567 w574 _] -> w368
      tunnel: w367 -> [_ _ w450 w553 w560 w567 w574 _]
      tunnel: w366 -> [_ _ w462 w554 w561 w568 w575 _]
      tunnel: [_ _ _ _ _ _ _ TRUE ("status")] -> w360
      tunnel: [_ w429 w456 w556 w563 w570 w577 _] -> w365
      tunnel: w362 -> [_ _ w456 w556 w563 w570 w577 w584]
      tunnel: [_ _ w454 w555 w562 w569 w576 _] -> w363
      tunnel: w364 -> [_ _ w463 w555 w562 w569 w576 _]
      frame "InitializeJoystick" {
        # "Initialize Joystick and Shutter Controls"
        n156 = property on="JoystOffset" class="Clust (strict)"() -> ("Value"=w376:T2)  [unwired: 2 in, 2 out]
        n157 = Bundle By Name(cluster=w376, "XOffset"=-99999, "YOffset"=-99999, "ZOffset"=-99999) -> (w378:T2)
        n158 = call <vilib>:"Initialize Joystick.vi"() -> ("device ID"=w377:refnum<k1>)  [unwired: 10 in, 1 out]
      }
      frame "InitializeMotors" {
        w382 = T1."BasicMode"
        w435 = 83829794  # Z Axis Controller ID
        w441 = 83829822  # Y Axis Controller ID
        w447 = 83829798  # X Axis Controller ID
        n159 = property on="IsActive?" class="Bool (strict)"(error in=w431, "Value"=FALSE ("IsYMotorActive?")) -> (error out=w442:errorcluster)  [unwired: 1 in, 1 out]
        n160 = property on="IsActive?" class="Bool (strict)"(error in=w431, "Value"=FALSE ("IsYMotorActive?")) -> (error out=w448:errorcluster)  [unwired: 1 in, 1 out]
        n161 = property on="IsActive?" class="Bool (strict)"(error in=w431, "Value"=FALSE ("IsYMotorActive?")) -> (error out=w436:errorcluster)  [unwired: 1 in, 1 out]
        n162 = call "s_InitializeMotor.vi"("Error In"=w442, "Servo Controller  ID"=w441, "Motor Reference In"="YMotorRef") -> ("Error Out"=w443:errorcluster, "Motor Reference"=w424:refnum<k7>)
        n163 = call "s_InitializeMotor.vi"("Error In"=w448, "Servo Controller  ID"=w447, "Motor Reference In"="XMotorRef") -> ("Error Out"=w449:errorcluster, "Motor Reference"=w428:refnum<k7>)
        n164 = call "s_InitializeMotor.vi"("Error In"=w436, "Servo Controller  ID"=w435, "Motor Reference In"="ZMotorRef") -> ("Error Out"=w437:errorcluster, "Motor Reference"=w421:refnum<k7>)
        n165 = property on="IsActive?" class="Bool (strict)"(error in=w443, "Value"=TRUE ("IsYMotorActive?")) -> (error out=w423:errorcluster)  [unwired: 1 in, 1 out]
        n166 = Unbundle By Name("Motor Limits") -> ("XMin"=w388:sgl, "XMax"=w387:sgl, "YMin"=w386:sgl, "YMax"=w385:sgl, "ZMin"=w384:sgl, "ZMax"=w383:sgl)
        n167 = property on="IsActive?" class="Bool (strict)"(error in=w449, "Value"=TRUE ("IsYMotorActive?")) -> (error out=w426:errorcluster)  [unwired: 1 in, 1 out]
        n168 = property on="IsActive?" class="Bool (strict)"(error in=w437, "Value"=TRUE ("IsYMotorActive?")) -> (error out=w420:errorcluster)  [unwired: 1 in, 1 out]
        n169 = invoke class="MG17Motor" method="SetStageAxisInfo"(reference=w428, error in=w426, "lChanID"=0, "fMinPos"=w388, "fMaxPos"=w387, "lUnits"=1, "fPitch"=sgl 1.0, "lDirSense"=0) -> (reference out=w419:refnum<k7>, error out=w418:errorcluster, "lChanID"=w417:i32)  [unwired: 1 in, 6 out]
        n170 = invoke class="MG17Motor" method="SetStageAxisInfo"(reference=w424, error in=w423, "lChanID"=0, "fMinPos"=w386, "fMaxPos"=w385, "lUnits"=1, "fPitch"=sgl 1.0, "lDirSense"=0) -> (reference out=w411:refnum<k7>, error out=w410:errorcluster, "lChanID"=w409:i32)  [unwired: 1 in, 6 out]
        n171 = invoke class="MG17Motor" method="SetStageAxisInfo"(reference=w421, error in=w420, "lChanID"=0, "fMinPos"=w384, "fMaxPos"=w383, "lUnits"=1, "fPitch"=sgl 1.0, "lDirSense"=0) -> (reference out=w406:refnum<k7>, error out=w405:errorcluster, "lChanID"=w404:i32)  [unwired: 1 in, 6 out]
        n172 = invoke class="MG17Motor" method="GetPosition_Position"(reference=w411, error in=w410, "lChanID"=w409) -> (reference out=w403:refnum<k7>, error out=w413:errorcluster, "GetPosition_Position"=w412:sgl)  [unwired: 1 in, 1 out]
        n173 = invoke class="MG17Motor" method="GetPosition_Position"(reference=w406, error in=w405, "lChanID"=w404) -> (reference out=w402:refnum<k7>, error out=w408:errorcluster, "GetPosition_Position"=w407:sgl)  [unwired: 1 in, 1 out]
        n174 = invoke class="MG17Motor" method="GetPosition_Position"(reference=w419, error in=w418, "lChanID"=w417) -> (reference out=w416:refnum<k7>, error out=w415:errorcluster, "GetPosition_Position"=w414:sgl)  [unwired: 1 in, 1 out]
        n175 = property on="Pos (mm)" class="DigNum (strict)"(error in=w413, "Value"=w412) -> (error out=w401:errorcluster)  [unwired: 1 in, 1 out]
        n176 = property on="Pos (mm)" class="DigNum (strict)"(error in=w408, "Value"=w407) -> (error out=w399:errorcluster)  [unwired: 1 in, 1 out]
        n177 = property on="Pos (mm)" class="DigNum (strict)"(error in=w415, "Value"=w414) -> (error out=w400:errorcluster)  [unwired: 1 in, 1 out]
        n178 = Bundle("Motor Reference"=w416, "Motor Reference"=w403, "Motor Reference"=w402) -> (w429:T13)  [unwired: 1 in]
        n179 = Merge Errors(w400, w401, w399) -> (w430:errorcluster)
        n180 = property on="InstrumentMode" class="Enum (strict)"("Value"=w382) -> ()  [unwired: 2 in, 2 out]
      }
      frame "BasicMode" {
        n181 = call-poly <vilib>:"Acquire Input Data.vi"("device ID"=w467, "error in (no error)"=w466) -> ("device ID 2"=w465:refnum<k1>, "axis info"=w461:T14, "button info"=w451:T15, "error out"=w452:errorcluster)  [unwired: 13 in, 1 out]
        n182 = call "j_GetJoystickSignal.vi"("RelJoyPos In"=w463, "NewJoystButtInfo"=w451, "NewJoystAxisInfo"=w461, "OldJoystButtInfo"=w450, "OldJoystickOffset"=w462) -> ("MoveZ"=→"Move Z":bool, "MoveXY"=→"Move XY":bool, "Joystick Offset"=w464:T2, "RelJoyPos"=w458:T3, "TalkToMotors?"=w455:bool)
        n183 = case shown="False" w455 {
          tunnel: w458 -> [w505 w509]
          tunnel: [w494 w526] -> w457
          tunnel: w456 -> [w504 w512]
          tunnel: w452 -> [w478 w511]
          tunnel: [w505 w509] -> w454
          frame False {
            # "Just Update Motor Position and Vel"
            n184 = Unbundle(w504) -> ("Motor Reference"=w503:refnum<k7>, "Motor Reference"=w496:refnum<k7>, "Motor Reference"=w495:refnum<k7>)
            n185 = property on="Pos (mm)" class="DigNum (strict)"(error in=w478) -> (error out=w486:errorcluster, "Value"=w483:sgl)  [unwired: 1 in, 1 out]
            n186 = property on="Pos (mm)" class="DigNum (strict)"(error in=w478) -> (error out=w479:errorcluster, "Value"=w476:sgl)  [unwired: 1 in, 1 out]
            n187 = property on="Pos (mm)" class="DigNum (strict)"(error in=w478) -> (error out=w487:errorcluster, "Value"=w492:sgl)  [unwired: 1 in, 1 out]
            n188 = invoke class="MG17Motor" method="GetPosition_Position"(reference=w496, error in=w486, "lChanID"=0) -> (error out=w499:errorcluster, "GetPosition_Position"=w484:sgl)  [unwired: 1 in, 2 out]
            n189 = invoke class="MG17Motor" method="GetPosition_Position"(reference=w495, error in=w479, "lChanID"=0) -> (error out=w497:errorcluster, "GetPosition_Position"=w475:sgl)  [unwired: 1 in, 2 out]
            n190 = property on="MotorLoopDelay" class="DigNum (strict)"() -> ("Value"=w471:u32)  [unwired: 2 in, 2 out]
            n191 = invoke class="MG17Motor" method="GetPosition_Position"(reference=w503, error in=w487, "lChanID"=0) -> (error out=w501:errorcluster, "GetPosition_Position"=w493:sgl)  [unwired: 1 in, 2 out]
            n192 = To Single Precision Float(number=w471) -> (single precision float=w470:sgl)
            n193 = Subtract(x=w493, y=w492) -> (x-y=w491:sgl)
            n194 = property on="Pos (mm)" class="DigNum (strict)"(error in=w499, "Value"=w484) -> (error out=w482:errorcluster)  [unwired: 1 in, 1 out]
            n195 = Subtract(x=w484, y=w483) -> (x-y=w485:sgl)
            n196 = Subtract(x=w475, y=w476) -> (x-y=w477:sgl)
            n197 = property on="Pos (mm)" class="DigNum (strict)"(error in=w497, "Value"=w475) -> (error out=w474:errorcluster)  [unwired: 1 in, 1 out]
            n198 = property on="Pos (mm)" class="DigNum (strict)"(error in=w501, "Value"=w493) -> (error out=w489:errorcluster)  [unwired: 1 in, 1 out]
            n199 = Divide(x=w470, y=sgl 1000.0) -> (x/y=w468:sgl)
            n200 = Divide(x=w491, y=w468) -> (x/y=w490:sgl)
            n201 = Divide(x=w485, y=w468) -> (x/y=w481:sgl)
            n202 = Divide(x=w477, y=w468) -> (x/y=w473:sgl)
            n203 = property on="Vel (mm/s)" class="DigNum (strict)"(error in=w489, "Value"=w490) -> (error out=w488:errorcluster)  [unwired: 1 in, 1 out]
            n204 = property on="Vel (mm/s)" class="DigNum (strict)"(error in=w482, "Value"=w481) -> (error out=w480:errorcluster)  [unwired: 1 in, 1 out]
            n205 = property on="Vel (mm/s)" class="DigNum (strict)"(error in=w474, "Value"=w473) -> (error out=w472:errorcluster)  [unwired: 1 in, 1 out]
            n206 = Merge Errors(w488, w480, w472) -> (w494:errorcluster)
          }
          frame True {
            # ">ZMotRef>"
            # ">YMotRef>"
            # ">XMotRef>"
            n207 = Unbundle By Name(w509) -> ("XRelPos"=w542:i32, "YRelPos"=w528:i32, "ZRelPos"=w513:i32)
            n208 = Unbundle(w512) -> ("Motor Reference"=w508:refnum<k7>, "Motor Reference"=w507:refnum<k7>, "Motor Reference"=w506:refnum<k7>)
            n209 = property on="Direction" class="DigNum (strict)"(error in=w511) -> (error out=w541:errorcluster, "Value"=w540:i32)  [unwired: 1 in, 1 out]
            n210 = property on="Direction" class="DigNum (strict)"(error in=w511) -> (error out=w531:errorcluster, "Value"=w530:i32)  [unwired: 1 in, 1 out]
            n211 = property on="Direction" class="DigNum (strict)"(error in=w511) -> (error out=w516:errorcluster, "Value"=w515:i32)  [unwired: 1 in, 1 out]
            n212 = property on="Move Z" class="Bool (strict)"(error in=w516) -> (error out=w524:errorcluster, "Value"=w523:bool)  [unwired: 1 in, 1 out]
            n213 = property on="Move XY" class="Bool (strict)"(error in=w541) -> (error out=w550:errorcluster, "Value"=w549:bool)  [unwired: 1 in, 1 out]
            n214 = property on="Move XY" class="Bool (strict)"(error in=w531) -> (error out=w539:errorcluster, "Value"=w538:bool)  [unwired: 1 in, 1 out]
            n215 = call "j_MotorExecute.vi"("MoveChamber?"=w549, "Axis Motor Settings"="X Motor Settings", "Error In"=w550, "JoystRelPos"=w542, "Motor's Old Direction"=w540, "Motor Reference In"=w508) -> ("Error Out"=w545:errorcluster, "Motor Position (mm)"=w544:sgl, "Motor's New Direction"=w543:i32, "Motor Velocity (mm/s)"=w546:sgl)  [unwired: 1 out]
            n216 = call "j_MotorExecute.vi"("MoveChamber?"=w538, "Axis Motor Settings"="Y Motor Settings", "Error In"=w539, "JoystRelPos"=w528, "Motor's Old Direction"=w530, "Motor Reference In"=w507) -> ("Error Out"=w534:errorcluster, "Motor Position (mm)"=w533:sgl, "Motor's New Direction"=w532:i32, "Motor Velocity (mm/s)"=w535:sgl)  [unwired: 1 out]
            n217 = call "j_MotorExecute.vi"("MoveChamber?"=w523, "Axis Motor Settings"="Z Motor Settings", "Error In"=w524, "JoystRelPos"=w513, "Motor's Old Direction"=w515, "Motor Reference In"=w506) -> ("Error Out"=w519:errorcluster, "Motor Position (mm)"=w518:sgl, "Motor's New Direction"=w517:i32, "Motor Velocity (mm/s)"=w520:sgl)  [unwired: 1 out]
            n218 = property on="Pos (mm)" class="DigNum (strict)"(error in=w545, "Value"=w544) -> (error out=w547:errorcluster)  [unwired: 1 in, 1 out]
            n219 = property on="Pos (mm)" class="DigNum (strict)"(error in=w534, "Value"=w533) -> (error out=w536:errorcluster)  [unwired: 1 in, 1 out]
            n220 = property on="Pos (mm)" class="DigNum (strict)"(error in=w519, "Value"=w518) -> (error out=w521:errorcluster)  [unwired: 1 in, 1 out]
            n221 = property on="Vel (mm/s)" class="DigNum (strict)"(error in=w547, "Value"=w546) -> (error out=w548:errorcluster)  [unwired: 1 in, 1 out]
            n222 = property on="Vel (mm/s)" class="DigNum (strict)"(error in=w536, "Value"=w535) -> (error out=w537:errorcluster)  [unwired: 1 in, 1 out]
            n223 = property on="Vel (mm/s)" class="DigNum (strict)"(error in=w521, "Value"=w520) -> (error out=w522:errorcluster)  [unwired: 1 in, 1 out]
            n224 = property on="Direction" class="DigNum (strict)"(error in=w537, "Value"=w532) -> (error out=w525:errorcluster)  [unwired: 1 in, 1 out]
            n225 = property on="Direction" class="DigNum (strict)"(error in=w548, "Value"=w543) -> (error out=w527:errorcluster)  [unwired: 1 in, 1 out]
            n226 = property on="Direction" class="DigNum (strict)"(error in=w522, "Value"=w517) -> (error out=w510:errorcluster)  [unwired: 1 in, 1 out]
            n227 = Merge Errors(w527, w525, w510) -> (w526:errorcluster)
          }
        }
        n228 = property on="InstrumentMode" class="Enum (strict)"() -> ("Value"=w453:T1)  [unwired: 2 in, 2 out]
      }
      frame "PassiveMode" {
        n229 = property on="InstrumentMode" class="Enum (strict)"() -> ("Value"=w558:T1)  [unwired: 2 in, 2 out]
      }
      frame "AcquireOffsetMode" {
        n230 = property on="InstrumentMode" class="Enum (strict)"() -> ("Value"=w565:T1)  [unwired: 2 in, 2 out]
      }
      frame "AcquireSpectrumMode" {
        n231 = property on="InstrumentMode" class="Enum (strict)"() -> ("Value"=w572:T1)  [unwired: 2 in, 2 out]
      }
      frame "Force-ExtensionMode" {
        n232 = property on="InstrumentMode" class="Enum (strict)"() -> ("Value"=w579:T1)  [unwired: 2 in, 2 out]
      }
      frame "Shutdown" {
        n233 = call-poly <vilib>:"Close Input Device.vi"("error in (no error)"=w583, "device ID"=w582) -> ("error out"=w591:errorcluster)  [unwired: 8 in]
        n234 = Unbundle(w584) -> ("Motor Reference"=w587:refnum<k7>, "Motor Reference"=w586:refnum<k7>, "Motor Reference"=w585:refnum<k7>)
        n235 = call "s_CloseMotor.vi"("Error In"=w591, "Motor Reference In"=w587) -> ("Error Out"=w596:errorcluster)
        n236 = call "s_CloseMotor.vi"("Error In"=w591, "Motor Reference In"=w586) -> ("Error Out"=w594:errorcluster)
        n237 = call "s_CloseMotor.vi"("Error In"=w591, "Motor Reference In"=w585) -> ("Error Out"=w592:errorcluster)
        n238 = property on="IsActive?" class="Bool (strict)"(error in=w596, "Value"=FALSE ("IsYMotorActive?")) -> (error out=w590:errorcluster)  [unwired: 1 in, 1 out]
        n239 = property on="IsActive?" class="Bool (strict)"(error in=w594, "Value"=FALSE ("IsYMotorActive?")) -> (error out=w589:errorcluster)  [unwired: 1 in, 1 out]
        n240 = property on="IsActive?" class="Bool (strict)"(error in=w592, "Value"=FALSE ("IsYMotorActive?")) -> (error out=w588:errorcluster)  [unwired: 1 in, 1 out]
        n241 = Merge Errors(w590, w589, w588) -> (w581:errorcluster)
        n242 = property on="InstrumentMode" class="Enum (strict)"(error in=w581) -> (error out=w580:errorcluster, "Value"=w598:T1)  [unwired: 1 in, 1 out]
      }
    }
  }
